vi "ReadAnalogArduino.vi"() -> ()   [LabVIEW 2015]
uses:
  <vilib>/MakerHub/LINX/Public/Peripherals/Analog/Analog Read 1 Chan.vi
  <vilib>/addons/control/pid/pid.llb/PID Control Input Filter (DBL).vi
  <vilib>/MakerHub/LINX/Public/Peripherals/Digital/Digital Write 1 Chan.vi
  <vilib>/MakerHub/LINX/LMH-LINX.lvlib
  <vilib>/addons/control/pid/NI_PID_pid.lvlib
panel:
  in  "flow meter type":enum16{"80", "1000", "5000"}(ring)
  out "Waveform Chart 2":dbl(graph)
  in  "80ul/min flow meter channel":u8=8
  in  "Valve Arduino Channel":u8
  in  "Valve Direction":bool
  in  "stop":bool
  in  "Analog Channel":u8
  in  "Serial Port":refnum<visa-resource-name>="N/A"
  out "Error Out":errorcluster
  in  "Error In":errorcluster
  out "Waveform Chart":dbl(graph)
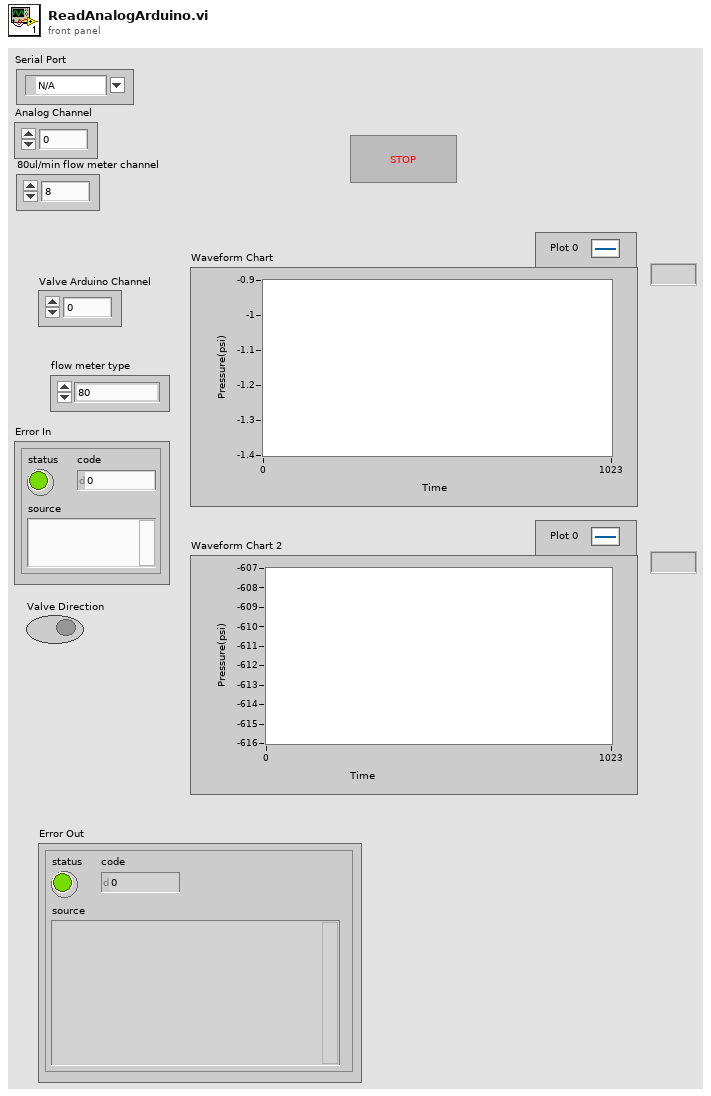
[diagram p1: front panel]
types:
  T1 = typedef "LMH-LINX.lvlib/LINX Ref.ctl" = cluster{"Platform":T2, "Interface":T3, "LINX Device Config":T4}
  T2 = typedef "LMH-LINX.lvlib/Platform.ctl" = enum16{"LINX", "myRIO"}
  T3 = typedef "LMH-LINX.lvlib/Interface.ctl" = enum16{"Serial", "TCP"}
  T4 = typedef "LMH-LINX.lvlib/Device.lvlib/LINX Device Config.ctl" = cluster{"Interface":T3, "COM Port":refnum<visa-resource-name>, "TCP Configuration":T5, "Device Family":u8, "Device ID":u8, "Device Name":string, "TCP Ref":refnum<k5>, "Channels":T6}
  T5 = typedef "LMH-LINX.lvlib/Device.lvlib/TCP Config.ctl" = cluster{"IP Address":string, "Port":u16}
  T6 = typedef "LMH-LINX.lvlib/Channels.ctl" = cluster{"DI":u8[], "DO":u8[], "AI":u8[], "AO":u8[], "PWM":u8[], "QE":u8[], "UART":u8[], "I2C 2":u8[], "SPI":u8[], "CAN":u8[], "Servo":u8[], "AI Ref (V)":dbl, "AO Ref (V)":dbl, "AO Resolution (Bits)":u8}
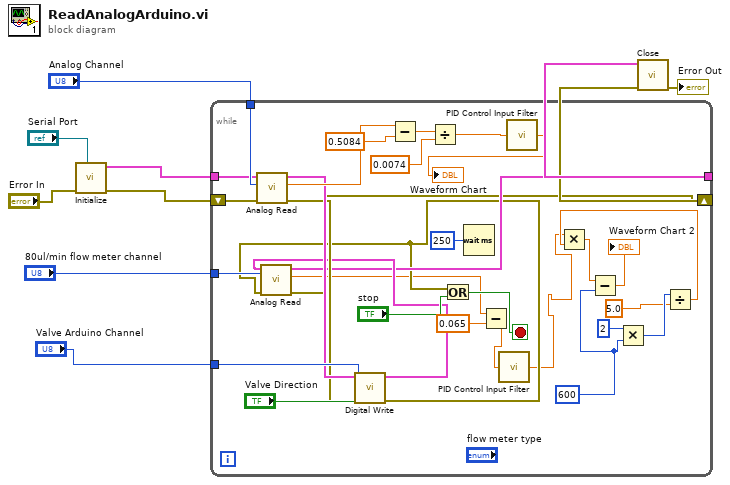
[diagram p0: block diagram]
diagram:
  n1 = call <vilib>:"Initialize.vi"("Serial Port"="Serial Port", "Error In"="Error In") -> ("Error Out"=w8:errorcluster, "LINX Ref"=w10:T1)  [unwired: 7 in, 1 out]
  n2 = while {
    shift-right: [w18] -> w7
    shift-left: w8 -> [w42]
    tunnel: w10 -> [w31]
    tunnel: [w26] -> w9
    tunnel: "Analog Channel" -> [w41]
    tunnel: "Valve Arduino Channel" -> [w32]
    tunnel: "80ul/min flow meter channel" -> [w28]
    stop <- w39 stop-if-true
    w17 = 600
    n3 = call-poly <vilib>:"Analog Read.vi"("Error In"=w42, "Analog Channel"=w41, "LINX Resource"=w31) -> ("Error Out"=w29:errorcluster, "AI Value"=w37:dbl, "LINX Resource"=w30:T1)  [unwired: 5 in, 1 out]
    n4 = call-poly <vilib>:"Digital Write.vi"("Error In"=w29, "Output Value"="Valve Direction", "DO Channel"=w32, "LINX Resource"=w30) -> ("Error Out"=w19:errorcluster, "LINX Resource"=w27:T1)  [unwired: 6 in]
    n5 = call-poly <vilib>:"Analog Read.vi"("Error In"=w19, "Analog Channel"=w28, "LINX Resource"=w27) -> ("Error Out"=w18:errorcluster, "AI Value"=w16:dbl, "LINX Resource"=w26:T1)  [unwired: 5 in, 1 out]
    n6 = Subtract(x=w37, y=0.5084) -> (x-y=w35:dbl)
    n7 = Divide(x=w35, y=0.0074) -> (x/y=w12:dbl)
    n8 = Or(x=w19, y="stop") -> (x .or. y?=w39:bool)
    n9 = Wait (ms)(milliseconds to wait=u32 250) -> ()  [unwired: 1 out]
    n10 = Subtract(x=w16, y=0.065) -> (x-y=w14:dbl)
    n11 = call-poly <vilib>:"PID Control Input Filter.vi"("input"=w14) -> ("output"=w13:dbl)  [unwired: 4 in]
    n12 = call-poly <vilib>:"PID Control Input Filter.vi"("input"=w12) -> ("output"=→"Waveform Chart":dbl)  [unwired: 4 in]
    n13 = Multiply(x=2, y=w17) -> (x*y=w24:i32)
    n14 = Divide(x=w24, y=5.0) -> (x/y=w22:dbl)
    n15 = Multiply(x=w13, y=w22) -> (x*y=w21:dbl)
    n16 = Subtract(x=w21, y=w17) -> (x-y=→"Waveform Chart 2":dbl)
  }
  n17 = call <vilib>:"Close.vi"("Error In"=w7, "LINX Resource"=w9) -> ("Error Out"=→"Error Out":errorcluster)  [unwired: 8 in, 1 out]
